vi "Rename.vi"(8 "error in (no error)":errorcluster, 9 "NewName":string, 10 "OldName":string, 11 "PLC_Module in":refnum<class "PLC_Module.lvclass">) -> (0 "error out":errorcluster, 3 "PLC_Module out":refnum<class "PLC_Module.lvclass">)   [LabVIEW 2025, in "PLC_Module.lvlib" / "PLC_Module.lvclass"]
uses:
  PLC_Module.lvclass
  PLC_Module.lvclass/PLC_Module.ctl
  Read Configuration.vi
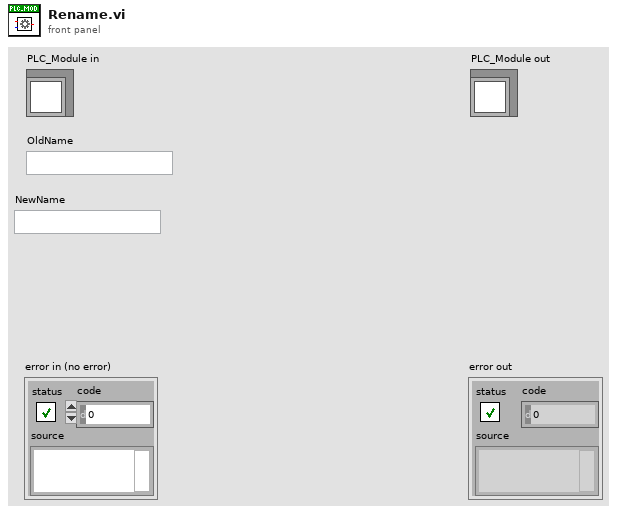
[diagram p1: front panel]
types:
  T1 = typedef "PLC_Module.lvlib/PLC_Module.lvclass/PLC_Data_Config.ctl" = map{string, cluster{"Config":T2, "Get Value":string, "Set Value":string}}
  T2 = typedef "PLC_Module.lvlib/PLC_Module.lvclass/PLC_Data.ctl" = cluster{"Address":string, "Direction":enum16{"PC->PLC", "PLC->PC"}, "DataType":T3, "Description":string}
  T3 = typedef "PLC_Module.lvlib/PLC_Module.lvclass/PLC_Data_Type.ctl" = enum16{"Boolean", "Single Float", "U8", "U32", "U32_Array", "String"}
  T4 = cluster{"Config":T2, "Get Value":string, "Set Value":string}
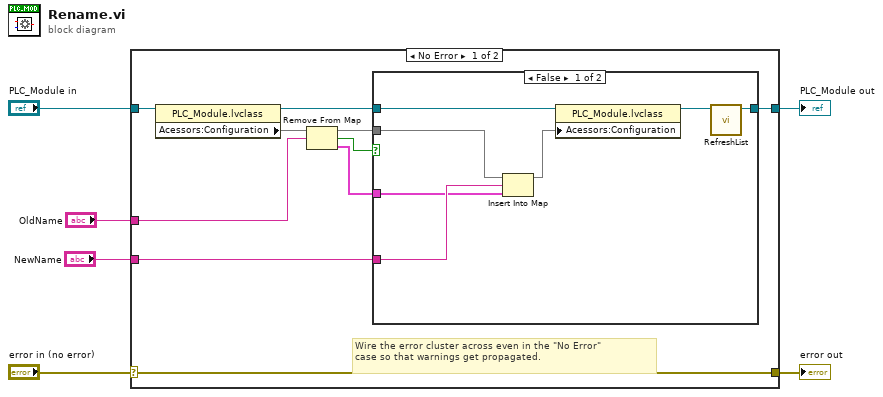
[diagram p0: block diagram]
diagram:
  n1 = case shown="No Error" "error in (no error)" {
    selector: "error in (no error)" -> [w15 w26]
    tunnel: [w15 w26] -> w5
    tunnel: [w9 w25] -> w3
    tunnel: "PLC_Module in" -> [w16 w25]
    tunnel: "OldName" -> [w13 _]
    tunnel: "NewName" -> [w11 _]
    frame No Error {
      # "Wire the error cluster across even in the \"No Error\"\ncase so that warnings get propagated."
      n2 = property class="PLC_Module.lvclass"(reference=w16) -> (reference out=w14:refnum<class "PLC_Module.lvclass">, "Acessors:Configuration"=w12:T1)  [unwired: 1 in, 1 out]
      n3 = Remove From Map(10:w13, 11:w12) -> (1:w10:T4, 2:w8:bool, 3:w7:T1)
      n4 = case shown="False" w8 {
        tunnel: w14 -> [w23 w24]
        tunnel: w7 -> [w22 _]
        tunnel: w11 -> [w21 _]
        tunnel: w10 -> [w20 _]
        tunnel: [w17 w24] -> w9
        frame False {
          n5 = Insert Into Map(map in=w22, key=w21, value=w20) -> (map out=w19:T1)  [unwired: 2 out]
          n6 = property class="PLC_Module.lvclass"(reference=w23, "Acessors:Configuration"=w19) -> (reference out=w18:refnum<class "PLC_Module.lvclass">)  [unwired: 1 in, 1 out]
          n7 = call "RefreshList.vi"("PLC_Module in"=w18) -> ("PLC_Module out"=w17:refnum<class "PLC_Module.lvclass">)  [unwired: 9 in, 1 out]
        }
        frame True {
        }
      }
    }
    frame Error {
    }
  }
  "error out" <- w5
  "PLC_Module out" <- w3
